vi "Get Report Path.vi"(8 "error in (no error)":errorcluster, 10 "parameters in":T1, 11 "Sequencer Module runtime in":refnum<class "Sequencer Module runtime.lvclass">) -> (0 "error out":errorcluster, 1 "Path":path, 2 "parameters out":T1, 3 "Sequencer Module runtime out":refnum<class "Sequencer Module runtime.lvclass">)   [LabVIEW 2015, in "Sequencer Module runtime.lvclass"]
uses:
  Sequencer Module runtime.lvclass
  <vilib>/NI/Tag Bus/table/data table.ctl
  Sequencer Module runtime.lvclass/Sequencer Module runtime.ctl
  <vilib>/NI/Tag Bus/table/data table.lvlib
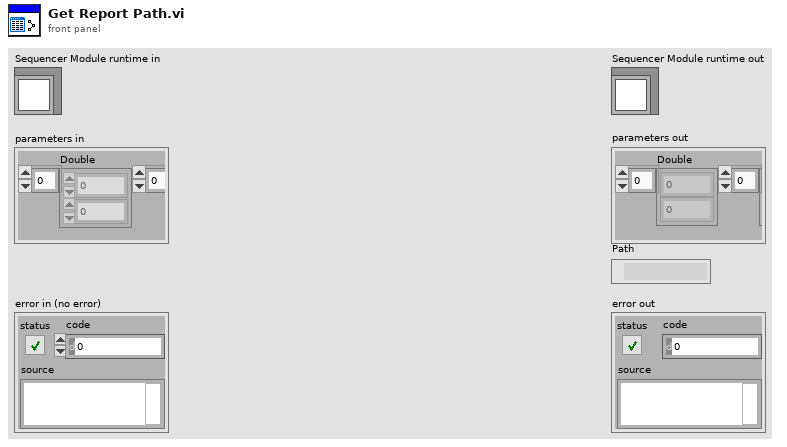
[diagram p1: front panel]
types:
  T1 = typedef "tag bus.lvlib/data table.lvlib/data table.ctl" = cluster{"Double":dbl[], "Single":sgl[], "I64":i64[], "I32":i32[], "I16":i16[], "I8":i8[], "U64":u64[], "U32":u32[], "U16":u16[], "U8":u8[], "Boolean":bool[], "String":string[], "Array of Double":cluster{"DBL Array":dbl[]}[], "Array of Single":cluster{"SGL Array":sgl[]}[], "Array of I64":cluster{"I64 Array":i64[]}[], "Array of I32":cluster{"I32 Array":i32[]}[], "Array of I16":cluster{"I16 Array":i16[]}[], "Array of I8":cluster{"I8 Array":i8[]}[], "Array of U64":cluster{"U64 Array":u64[]}[], "Array of U32":cluster{"U32 Array":u32[]}[], "Array of U16":cluster{"U16 Array":u16[]}[], "Array of U8":cluster{"U8 Array":u8[]}[], "Array of Boolean":cluster{"Boolean Array":bool[]}[], "Array of String":cluster{"String Array":string[]}[]}
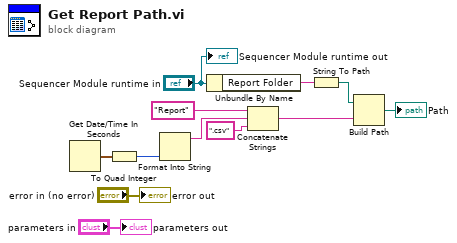
[diagram p0: block diagram]
diagram:
  n1 = Get Date/Time In Seconds() -> (seconds since 1Jan1904=w5:timestamp)
  n2 = To Quad Integer(1:w5) -> (0:w7:i64)
  n3 = Format Into String(w7) -> (resulting string=w6:string)  [unwired: 3 in, 1 out]
  n4 = Unbundle By Name("Sequencer Module runtime in") -> ("Report Folder"=w3:string)
  n5 = Concatenate Strings("Report" ("string"), w6, ".csv" ("string")) -> (w2:string)
  n6 = String To Path(string=w3) -> (path=w4:path)
  n7 = Build Path(base path=w4, name or relative path=w2) -> (appended path=→"Path":path)
  "error out" <- "error in (no error)"
  "parameters out" <- "parameters in"
  "Sequencer Module runtime out" <- "Sequencer Module runtime in"
